vi "DB_SelectCount.vi"(8 "error in (no error)":errorcluster, 11 "SQLite Connection in":refnum<class "Connection.lvclass">) -> (0 "error out":errorcluster, 1 "Array - Numeric":dbl[](array[numeric]), 3 "SQLite Connection":refnum<class "Connection.lvclass">)   [LabVIEW 2020]
uses:
  <vilib>/drjdpowell/SQLite Library/SQL Connection/Connection.lvclass
  <vilib>/drjdpowell/SQLite Library/SQL Statement/SQL Statement.lvclass/SQL Statement.ctl
  <vilib>/drjdpowell/SQLite Library/SQL Statement/Column I64.vi
  <vilib>/drjdpowell/SQLite Library/SQL Statement/Error Message.vi
  <vilib>/drjdpowell/SQLite Library/SQL Statement/SQL Statement.lvclass
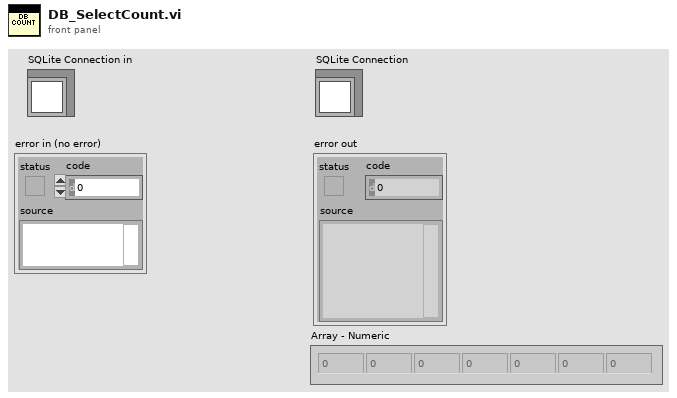
[diagram p1: front panel]
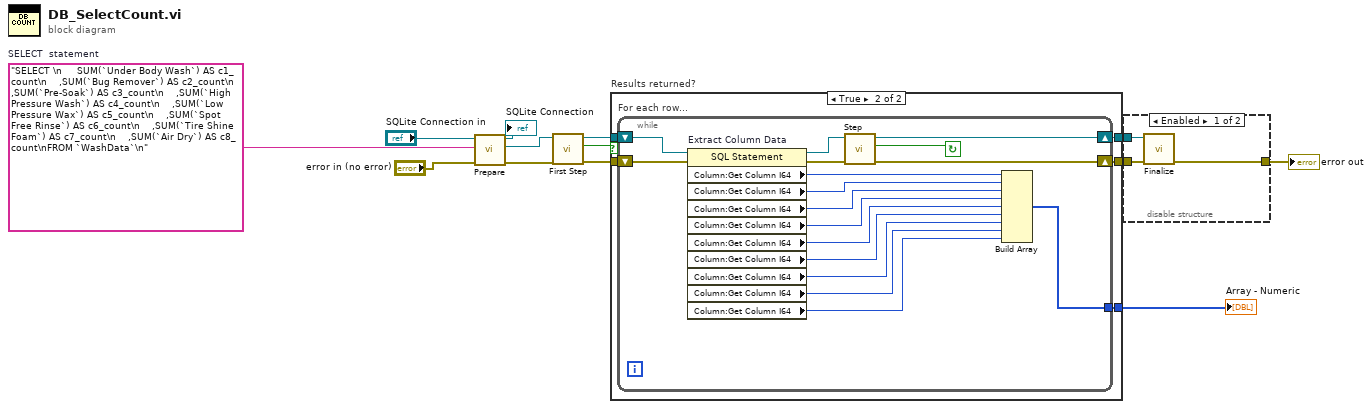
[diagram p0: block diagram]
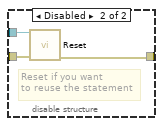
[diagram p2: hidden frame]
diagram:
  w11 = "SELECT \n     SUM(`Under Body Wash`) AS c1_count\n    ,SUM(`Bug Remover`) AS c2_count\n    ,SUM(`Pre-Soak`) AS c3_count\n    ,SUM(`High Pressure Wash`) AS c4_count\n    ,SUM(`Low Pressure Wax`) AS c5_count\n    ,SUM(`Spot Free Rinse`) AS c6_count\n    ,SUM(`Tire Shine Foam`) AS c7_count\n    ,SUM(`Air Dry`) AS c8_count\nFROM `WashData`\n"  # SELECT  statement
  n1 = call <vilib>:"Prepare.vi"("error in (no error)"="error in (no error)", "SQL"=w11, "SQLite Connection in"="SQLite Connection in") -> ("error out"=w7:errorcluster, "SQL Statement"=w6:refnum<class "SQL Statement.lvclass">, "SQLite Connection"=→"SQLite Connection":refnum<class "Connection.lvclass">)  [unwired: 4 in, 2 out]
  n2 = call <vilib>:"First Step.vi"("error in (no error)"=w7, "SQL Statement in"=w6) -> ("error out"=w9:errorcluster, "Row returned"=w8:bool, "SQL Statement"=w10:refnum<class "SQL Statement.lvclass">)  [unwired: 7 in]
  n3 = case "Results returned?" shown="True" w8 {
    tunnel: [w15 w20] -> w12
    tunnel: [w14 w19] -> w13
    tunnel: w10 -> [w15 w18]
    tunnel: w9 -> [w14 w17]
    tunnel: [_ w16] -> w1
    frame False {
    }
    frame True {
      n4 = while "For each row..." {
        shift-right: [w36] -> w20
        shift-left: w18 -> [w33]
        shift-right: [w34] -> w19
        shift-left: w17 -> [w32]
        tunnel: [w28] -> w16
        stop <- w31 continue-if-true
        n5 = property on="Extract Column Data" class="SQL Statement"(reference=w33, error in=w32) -> (reference out=w37:refnum<class "SQL Statement.lvclass">, error out=w35:errorcluster, "Column:Get Column I64"=w30:i64, "Column:Get Column I64"=w29:i64, "Column:Get Column I64"=w27:i64, "Column:Get Column I64"=w26:i64, "Column:Get Column I64"=w25:i64, "Column:Get Column I64"=w24:i64, "Column:Get Column I64"=w23:i64, "Column:Get Column I64"=w22:i64, "Column:Get Column I64"=w21:i64)
        n6 = call <vilib>:"Step.vi"("error in (no error)"=w35, "SQL Statement in"=w37) -> ("error out"=w34:errorcluster, "Row returned"=w31:bool, "SQL Statement"=w36:refnum<class "SQL Statement.lvclass">)  [unwired: 7 in]
        n7 = Build Array(w30, w29, w27, w26, w25, w24, w23, w22, w21) -> (w28:i64[])
      }
    }
  }
  "Array - Numeric" <- w1
  n8 = disable-structure "Diagram Disable Structure" shown="Enabled" {
    disable-tunnel: w12 -> [w40 w43]
    disable-tunnel: w13 -> [w39 w42]
    disable-tunnel: [w38 w41] -> w3
    frame Enabled {
      n9 = call <vilib>:"Finalize.vi"("error in (no error)"=w39, "SQL Statement in"=w40) -> ("error out"=w38:errorcluster)  [unwired: 9 in]
    }
    frame Disabled {
      # "Reset if you want\nto reuse the statement"
      n10 = call <vilib>:"Reset.vi"("error in (no error)"=w42, "SQL Statement in"=w43) -> ("error out"=w41:errorcluster)  [unwired: 8 in, 1 out]
    }
  }
  "error out" <- w3
